vi "Global_Vision_Data.vi"() -> ()   [LabVIEW 2017]
uses:
  TypeDefs/CLUST_Targeting Data.ctl
  TypeDefs/CLUST_Cube Data.ctl
  TypeDefs/CLUST_Road Navigation Data.ctl
  Systems/VisionHW Folder/VisionHW.lvlib
panel:
  in  "Targeting Data":T1
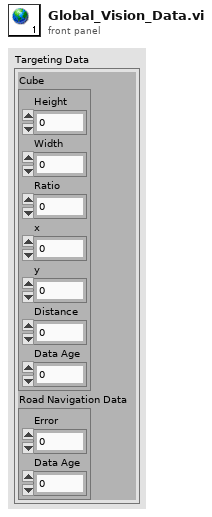
[diagram p1: front panel]
types:
  T1 = typedef "VisionHW.lvlib/CLUST_Targeting Data.ctl" = cluster{"Cube ":T2, "Road Navigation Data":T3}
  T2 = typedef "VisionHW.lvlib/CLUST_Cube Data.ctl" = cluster{"Height":dbl, "Width":dbl, "Ratio":dbl, "x":i32, "y":i32, "Distance ":i32, "Data Age":dbl}
  T3 = typedef "VisionHW.lvlib/CLUST_Road Navigation Data.ctl" = cluster{"Error":i32, "Data Age":dbl}
diagram:
